vi "Image.vi"(7 "JPG":refnum<vi>, 10 "queueName":string="PV_script", 11 "Console Reference":refnum<vi>) -> ()   [LabVIEW 2024]
uses:
  <vilib>/Utility/file.llb/Write Delimited Spreadsheet (DBL).vi
panel:
  in  "start":bool
  in  "Save":bool
  in  "python":string
  in  "Send":bool
  in  "Clear":bool
  in  "Tab Control":enum32{"Scope", "XY Plot", "Gauges"}(tab)
  out "Graph":dbl[][](graph)
  out "XY Plot":cluster{dbl[], dbl[]}[](graph)
  out "Gauge":dbl[](array[knob]) scale=-100.0..100.0
  out "Last Line":string
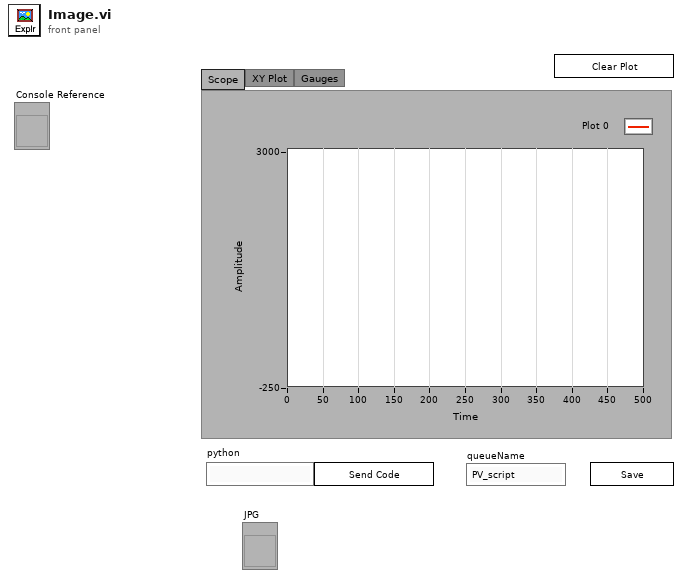
[diagram p1: front panel]
types:
  T1 = enum16{"Not data", "single values", "XY pairs", "Arrays", "Matrix"}
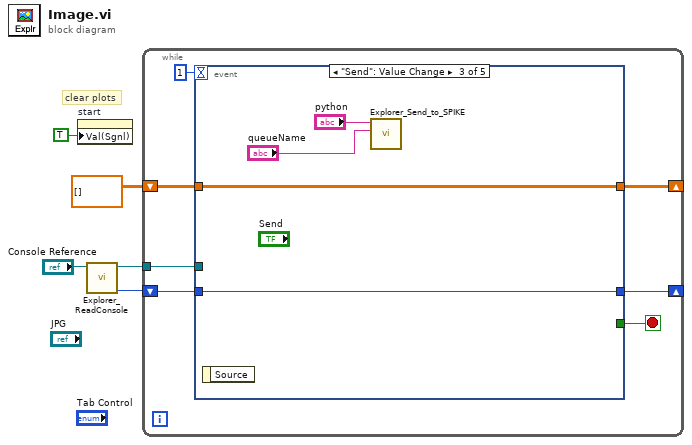
[diagram p0: block diagram]
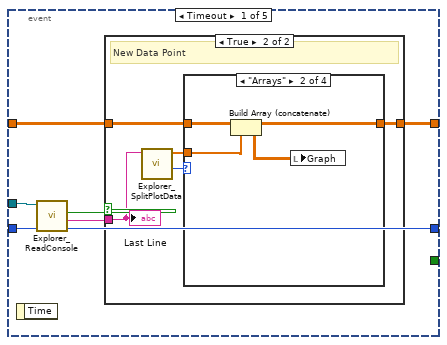
[diagram p2: hidden frame]
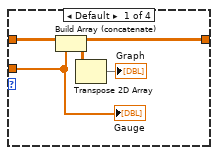
[diagram p4: hidden frame]
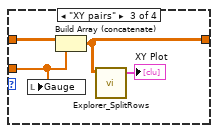
[diagram p5: hidden frame]
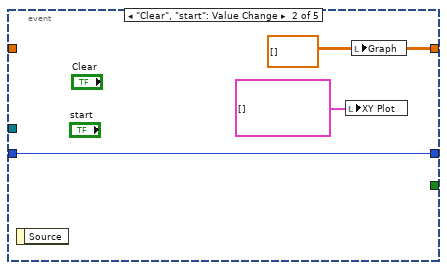
[diagram p7: hidden frame]
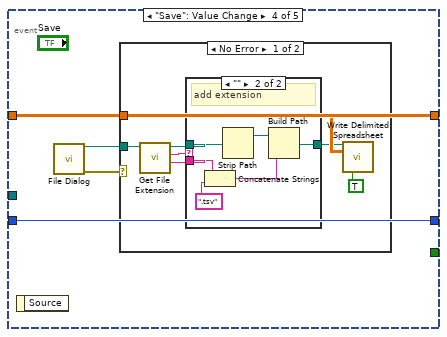
[diagram p8: hidden frame]
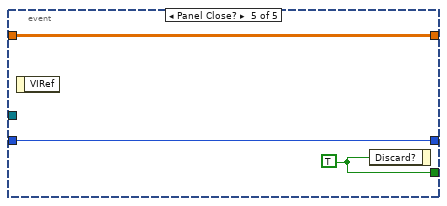
[diagram p11: hidden frame]
diagram:
  # "clear plots"
  n1 = property on="start" class="Bool (strict)"("Val(Sgnl)"=TRUE ("Value (Signaling)")) -> ()  [unwired: 2 in, 2 out]
  n2 = call "Explorer_ReadConsole.vi"("String in"="Console Reference") -> ("index out"=w4:i32, "String out"=w3:refnum<vi>)  [unwired: 6 in, 3 out]
  n3 = while {
    shift-right: [w10] -> _
    shift-left: w4 -> [w9]
    shift-right: [w7] -> _
    shift-left: dbl[][] [] -> [w8]
    tunnel: w3 -> [w6]
    stop <- w11 stop-if-true
    n4 = event shown="[2] \"Send\": Value Change" {
      selector: _ -> [_ _ _ _ _]
      dyn-events: _ -> [_ _ _ _ _]
      timeout: 1 -> [_ _ _ _ _]
      tunnel: [_ _ _ _ w65] -> w11
      tunnel: [w16 w40 w43 w48 w64] -> w10
      tunnel: w9 -> [w17 w40 w43 w48 w64]
      tunnel: w8 -> [w19 _ w44 w47 w63]
      tunnel: [w18 w39 w44 w47 w63] -> w7
      tunnel: w6 -> [w13 _ _ _ _]
      event Timeout {
        n5 = event-data() -> ()  [unwired: 1 in, 1 out]
        n6 = call "Explorer_ReadConsole.vi"("index in"=w17, "String in"=w13) -> ("index out"=w16:i32, "New Line"=w15:string, "New point?"=w14:bool)  [unwired: 5 in, 2 out]
        n7 = case shown="True" w14 {
          tunnel: w15 -> [_ w25]
          tunnel: w19 -> [w20 w24]
          tunnel: [w20 w23] -> w18
          frame False {
            # "nothing new"
          }
          frame True {
            # "New Data Point"
            n8 = call "Explorer_SplitPlotData.vi"("Value"=w25) -> ("Data type"=w22:T1, "Array"=w21:dbl[])  [unwired: 8 in, 1 out]
            n9 = case shown="\"Arrays\"" w22 {
              tunnel: w24 -> [w29 w32 w36 w37]
              tunnel: [w28 w30 w35 w37] -> w23
              tunnel: w21 -> [w26 w31 w33 _]
              frame Default {
                n10 = Build Array (concatenate)(w29, w26) -> (w28:dbl[][])
                n11 = Transpose 2D Array(2D array=w28) -> (transposed array=→"Graph":dbl[][])
                "Gauge" <- w26
              }
              frame "Arrays" {
                n12 = Build Array (concatenate)(w32, w31) -> (w30:dbl[][])
                n13 = local write "Graph"(w30) -> ()
              }
              frame "XY pairs" {
                n14 = local write "Gauge"(w33) -> ()
                n15 = Build Array (concatenate)(w36, w33) -> (w35:dbl[][])
                n16 = call "Explorer_SplitRows.vi"("Array in"=w35) -> ("XY Plot"=→"XY Plot":cluster{dbl[], dbl[]}[])  [unwired: 10 in]
              }
              frame "Not data" {
              }
            }
            "Last Line" <- w25
          }
        }
      }
      event "Clear", "start": Value Change {
        w39 = dbl[][] []
        n17 = event-data() -> ()  [unwired: 1 in, 1 out]
        n18 = local write "XY Plot"(cluster{dbl[], dbl[]}[] [] ("XY Plot")) -> ()
        n19 = local write "Graph"(w39) -> ()
      }
      event "Send": Value Change {
        n20 = event-data() -> ()  [unwired: 1 in, 1 out]
        n21 = call "Explorer_Send_to_SPIKE.vi"("queueName"="queueName", "python"="python") -> ()  [unwired: 9 in, 1 out]
      }
      event "Save": Value Change {
        n22 = event-data() -> ()  [unwired: 1 in, 1 out]
        n23 = call "File Dialog"() -> ("selected path"=w46:path, "error out"=w45:errorcluster)  [unwired: 12 in, 2 out]
        n24 = case shown="No Error" w45 {
          tunnel: w47 -> [w55 _]
          tunnel: w46 -> [w53 _]
          frame No Error {
            n25 = call <vilib>:"Get File Extension.vi"("file"=w53) -> ("filename without extension"=w49:string, "lowercase file extension"=w52:string, "dup file"=w50:path)  [unwired: 6 in, 2 out]
            n26 = case shown="\"\"" w52 {
              tunnel: [w56 w58] -> w51
              tunnel: w50 -> [w56 w60]
              tunnel: w49 -> [_ w62]
              frame Default {
              }
              frame "" {
                # "add extension"
                n27 = Concatenate Strings(w62, ".tsv" ("pattern (all files)")) -> (w57:string)
                n28 = Strip Path(path=w60) -> (stripped path=w59:path)  [unwired: 1 out]
                n29 = Build Path(base path=w59, name or relative path=w57) -> (appended path=w58:path)
              }
            }
            n30 = call-poly <vilib>:"Write Delimited Spreadsheet.vi"("file path (dialog if empty)"=w51, "2D data"=w55, "transpose? (no:F)"=TRUE) -> ()  [unwired: 11 in, 2 out]
          }
          frame Error {
          }
        }
      }
      event Panel Close? {
        w65 = TRUE ("Discard?")
        n31 = event-data() -> ()  [unwired: 1 in, 1 out]
        n32 = event-data("Discard?"=w65) -> ()  [unwired: 1 in, 1 out]
      }
    }
  }
